vi "fgt get pressure.vi"(8 "error in (no error)":errorcluster, 11 "pressureIndex":u32) -> (0 "error out":errorcluster, 3 "pressure out":sgl)   [LabVIEW 2020, in "fgt_SDK.lvlib"]
doc: "Read pressure value of selected device"
uses:
  fgt_SDK.lvlib
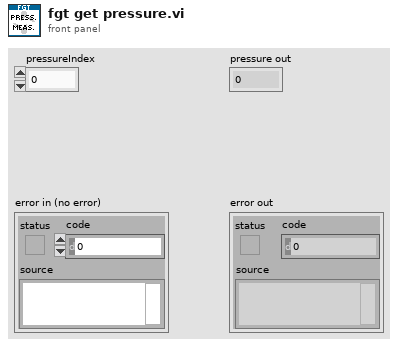
[diagram p1: front panel]
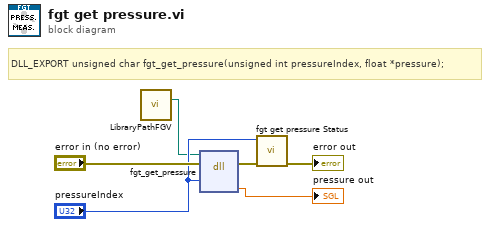
[diagram p0: block diagram]
diagram:
  # "DLL_EXPORT unsigned char fgt_get_pressure(unsigned int pressureIndex, float *pressure);"
  n1 = call "LibraryPathFGV.vi"() -> ("Path Out"=w1:path)  [unwired: 14 in, 1 out]
  n2 = dll-call lib="C:/Workspace/fgt-SDK/LabVIEW/dlls/fgt_SDK_*.*" fn="fgt_get_pressure"(path in=w1, error in="error in (no error)", "pressureIndex"="pressureIndex") -> (error out=w4:errorcluster, "pressure"=→"pressure out":sgl)  [unwired: 4 in, 1 out]
  n3 = call "fgt get pressure Status.vi"("error in (no error)"=w4, "pressureIndex"="pressureIndex") -> ("error out"=→"error out":errorcluster)  [unwired: 9 in]
